vi "通讯.vi"() -> ()   [LabVIEW 2016, in "斯坦道氨氮.lvlib"]
uses:
  <vilib>/Utility/config.llb/Write Key (String).vi
  <vilib>/Plasmionique/MB Master/MB_Master/MB_Master.lvclass
  <vilib>/Utility/config.llb/NI_LVConfig.lvlib
  <vilib>/Plasmionique/MB Master/MB Master.lvlib
panel:
  out "测量数据区":T1 {"单位" items=["ug/L", "mg/L", "ppm", "mg/m3", "cm", "ppb", "ug/m3", "%", "nmol/mol", "umol/mol", "MPN/L", "MPN/100ml", "ng/m3", "NTU", "无量纲", "ms/cm", "us/cm", "℃", "mV", "万个/L"]}
  out "状态告警区":u16[](array[numeric])
  out "测量数据区":u16[](array[numeric])
  out "序列号":string
  out "状态告警区":T2
  out "status":bool
  out "关键参数区":T3
  in  "读关键参数区":bool
  in  "读状态告警区":bool
  in  "读测量数据区":bool
  in  "站号":u16(ring) items=["总磷"=1, "氨氮"=3]
  in  "停止":bool
  in  "启动":bool
  in  "控制命令":u16(ring) items=["启动测量"=1, "标样核查"=2, "零点核查"=3, "跨度核查"=4, "空白测试"=5, "平行样测试"=6, "加标回收"=7, "空白校准"=8, "标样校准"=9, "初始化（清洗）"=10, "停止测试"=11, "仪器重启"=12, "校时"=13, "模式设置"=14, "测量间隔设置"=15]
  in  "控制命令参数":u16[](array[numeric]) format="%04xH"
  in  "VISA Resource":refnum<visa-resource-name>
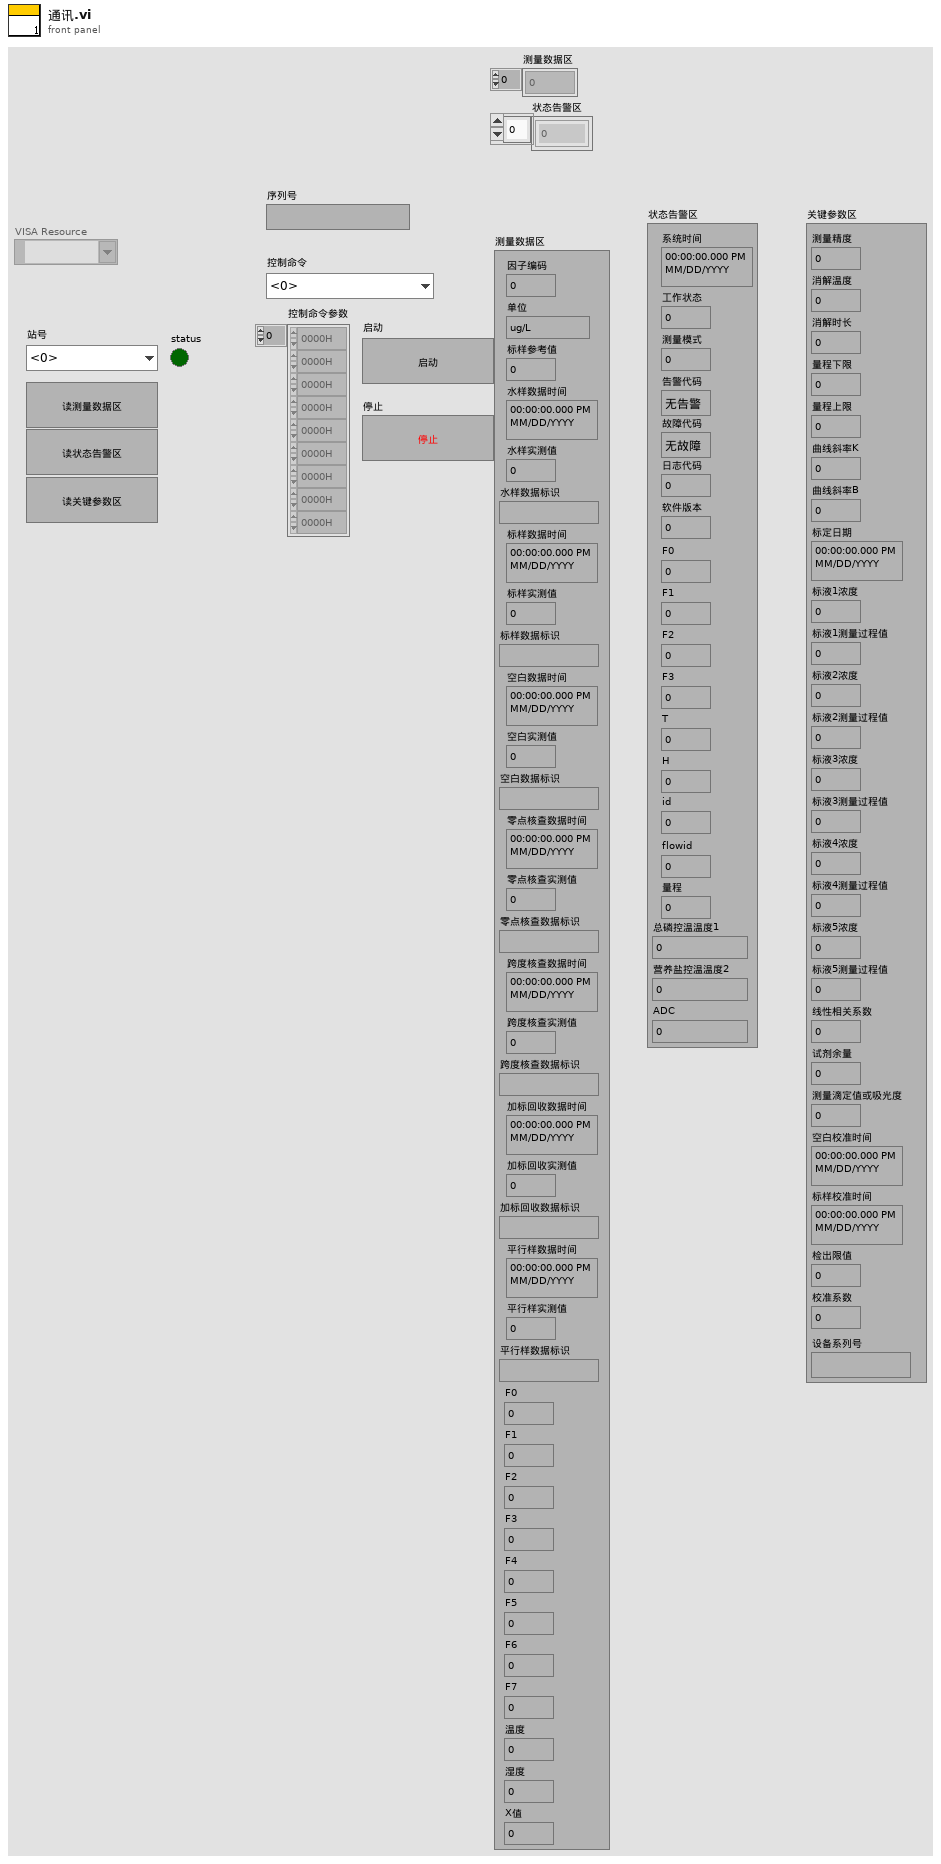
[diagram p1: front panel]
types:
  T1 = cluster{"因子编码":u32, "单位":u16, "标样参考值":sgl, "水样数据时间":timestamp, "水样实测值":sgl, "水样数据标识":string, "标样数据时间":timestamp, "标样实测值":sgl, "标样数据标识":string, "空白数据时间":timestamp, "空白实测值":sgl, "空白数据标识":string, "零点核查数据时间":timestamp, "零点核查实测值":sgl, "零点核查数据标识":string, "跨度核查数据时间":timestamp, "跨度核查实测值":sgl, "跨度核查数据标识":string, "加标回收数据时间":timestamp, "加标回收实测值":sgl, "加标回收数据标识":string, "平行样数据时间":timestamp, "平行样实测值":sgl, "平行样数据标识":string, "F0":sgl, "F1":sgl, "F2":sgl, "F3":sgl, "F4":sgl, "F5":sgl, "F6":sgl, "F7":sgl, "温度":sgl, "湿度":sgl, "X值":sgl}
  T2 = cluster{"系统时间":timestamp, "工作状态":u16, "测量模式":u16, "告警代码":enum16{"无告警", "缺试剂告警", "缺水样告警", "缺蒸馏水告警", "缺标液告警", "仪表漏液告警", "标定异常告警", "超量程告警", "加热异常", "低试剂预警", "超上限告警", "超下限告警", "仪表内部其他异常", "滴定异常告警", "电极异常告警", "量程切换告警", "参数设置告警", "PH电极电位异常", "电导率电极异常", "浊度光度异常", "溶解氧电极异常", "溶解氧光强异常", "温度异常告警", "PH异常告警", "溶解氧异常告警", "电导率异常告警", "浊度异常告警", "叶绿素异常告警", "藻密度异常告警", "蓝绿藻异常告警", "ORP异常告警", "氨氮异常告警", "清洁刷异常告警", "SD卡异常告警", "蓝牙异常告警", "Wifi异常告警", "流程异常告警"}, "故障代码":enum16{"无故障", "电机故障", "温度故障", "通讯故障", "滴定故障"}, "日志代码":u16, "软件版本":u16, "F0":sgl, "F1":sgl, "F2":sgl, "F3":sgl, "T":sgl, "H":sgl, "id":u16, "flowid":u16, "量程":u16, "ADC":sgl, "营养盐控温温度2":sgl, "总磷控温温度1":sgl}
  T3 = cluster{"测量精度":u16, "消解温度":u16, "消解时长":u16, "量程下限":sgl, "量程上限":sgl, "曲线斜率K":sgl, "曲线斜率B":sgl, "标定日期":timestamp, "标液1浓度":sgl, "标液1测量过程值":sgl, "标液2浓度":sgl, "标液2测量过程值":sgl, "标液3浓度":sgl, "标液3测量过程值":sgl, "标液4浓度":sgl, "标液4测量过程值":sgl, "标液5浓度":sgl, "标液5测量过程值":sgl, "线性相关系数":sgl, "试剂余量":u32, "测量滴定值或吸光度":sgl, "空白校准时间":timestamp, "标样校准时间":timestamp, "检出限值":sgl, "校准系数":sgl, "设备系列号":string}
  T4 = typedef "NI_LVConfig.lvlib/Config Data RefNum.ctl" = refnum<k1>
  T5 = enum8{"Enabled", "Disabled", "Disabled and Grayed Out"}
  T6 = cluster{"系统时间":timestamp, "工作状态":enum16{"空闲", "水样测试", "标样核查", "零点核查", "跨度核查", "空白测试", "平行样测试", "加标回收", "空白校准", "标样校准", "初始化（清洗）"}, "测量模式":enum16{"待机", "连续模式", "周期模式", "定点模式", "受控模式", "手动模式"}, "告警代码":enum16{"无告警", "缺试剂告警", "缺水样告警", "缺蒸馏水告警", "缺标液告警", "仪表漏液告警", "标定异常告警", "超量程告警", "加热异常", "低试剂预警", "超上限告警", "超下限告警", "仪表内部其他异常", "滴定异常告警", "电极异常告警", "量程切换告警", "参数设置告警", "PH电极电位异常", "电导率电极异常", "浊度光度异常", "溶解氧电极异常", "溶解氧光强异常", "温度异常告警", "PH异常告警", "溶解氧异常告警", "电导率异常告警", "浊度异常告警", "叶绿素异常告警", "藻密度异常告警", "蓝绿藻异常告警", "ORP异常告警", "氨氮异常告警", "清洁刷异常告警", "SD卡异常告警", "蓝牙异常告警", "Wifi异常告警", "流程异常告警"}, "故障代码":enum16{"无故障", "电机故障", "温度故障", "通讯故障", "滴定故障"}, "日志代码":u16, "软件版本":u16, "F0":sgl, "F1":sgl, "F2":sgl, "F3":sgl, "T":sgl, "H":sgl, "id":u16, "flowid":u16, "量程":u16, "总磷控温温度1":sgl, "营养盐控温温度2":sgl, "ADC":sgl}
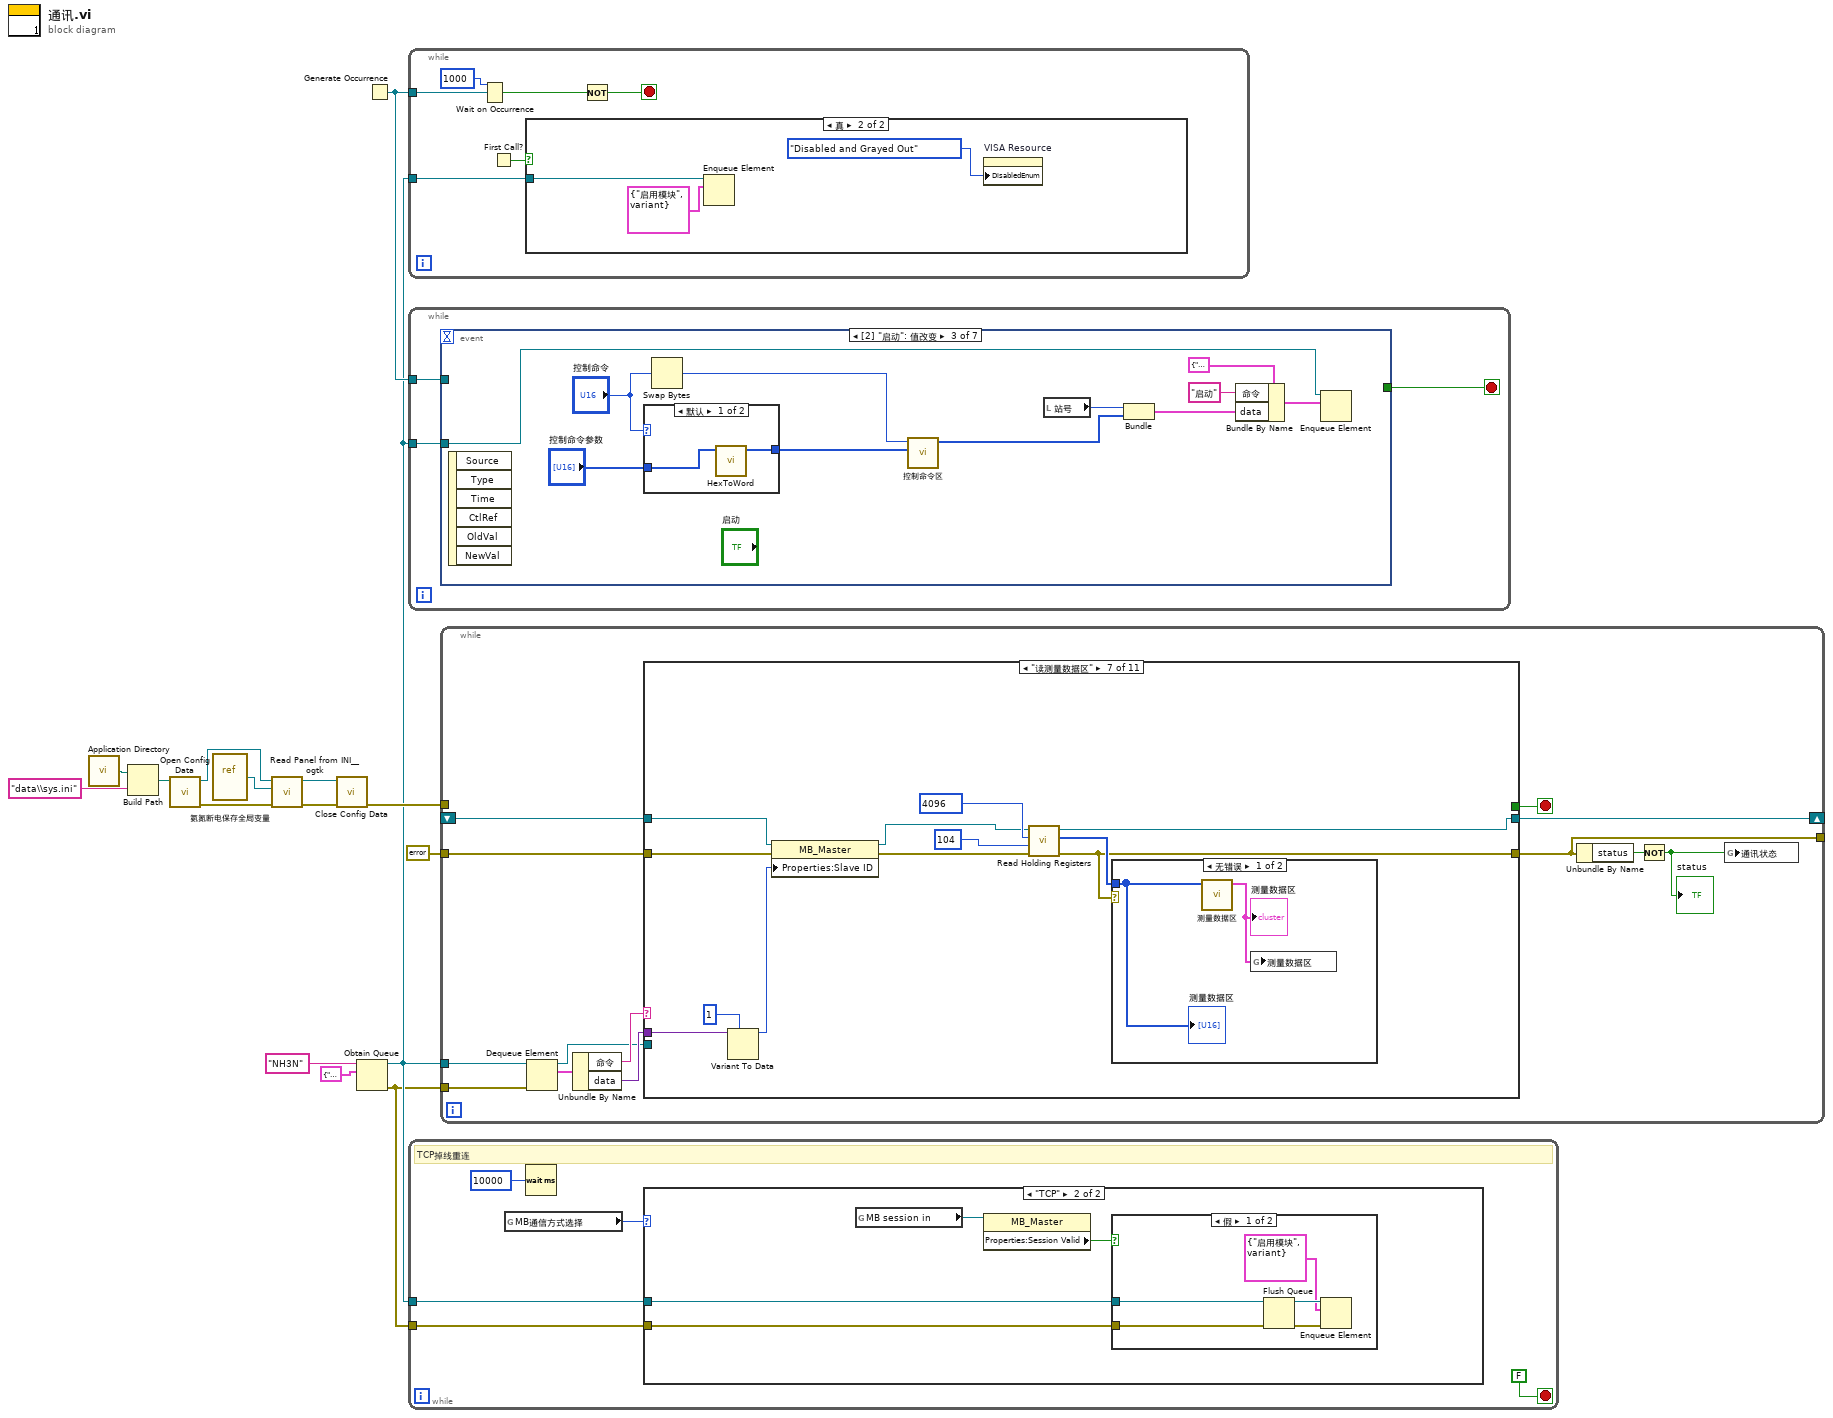
[diagram p0: block diagram]
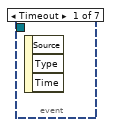
[diagram p5: hidden frame]
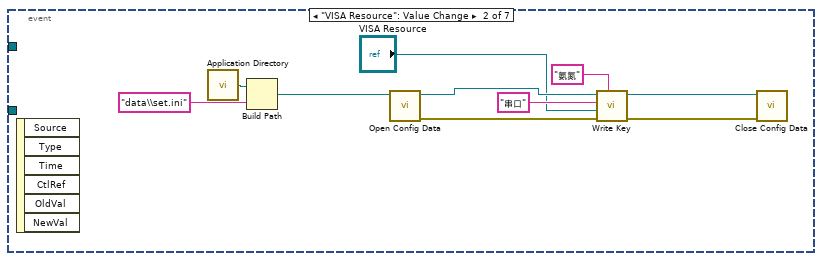
[diagram p6: hidden frame]
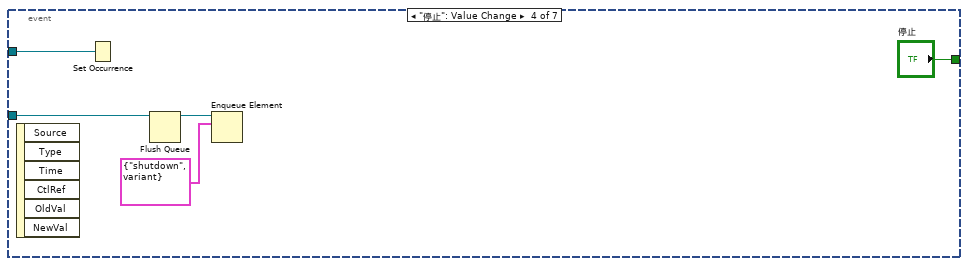
[diagram p8: hidden frame]
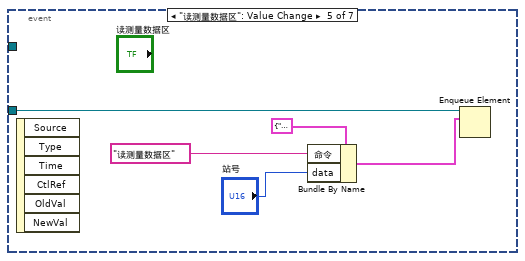
[diagram p9: hidden frame]
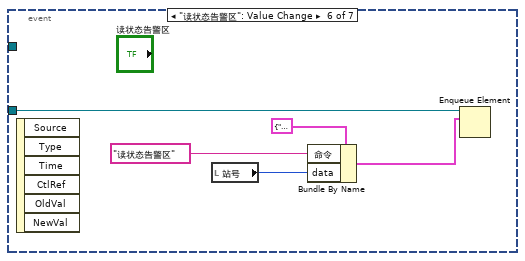
[diagram p10: hidden frame]
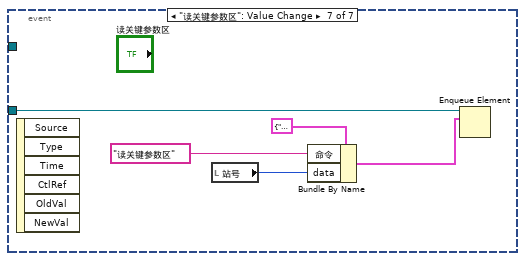
[diagram p11: hidden frame]
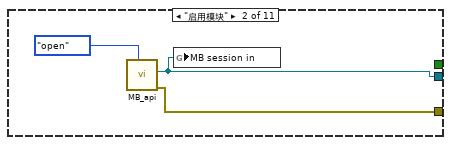
[diagram p13: hidden frame]
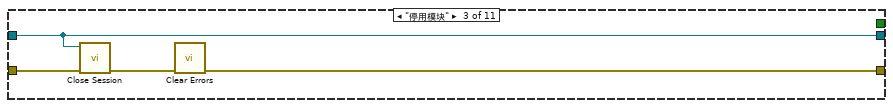
[diagram p14: hidden frame]
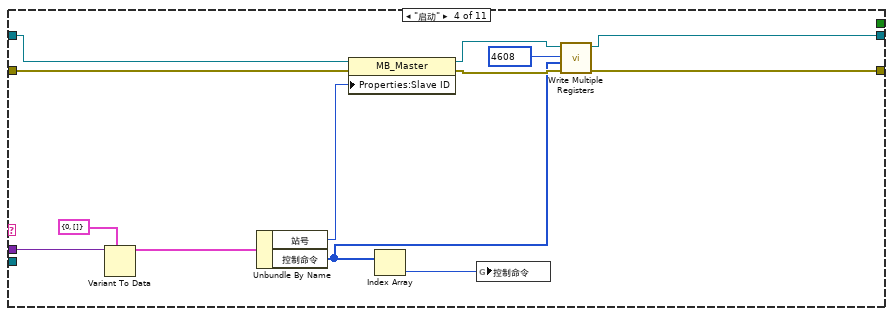
[diagram p15: hidden frame]
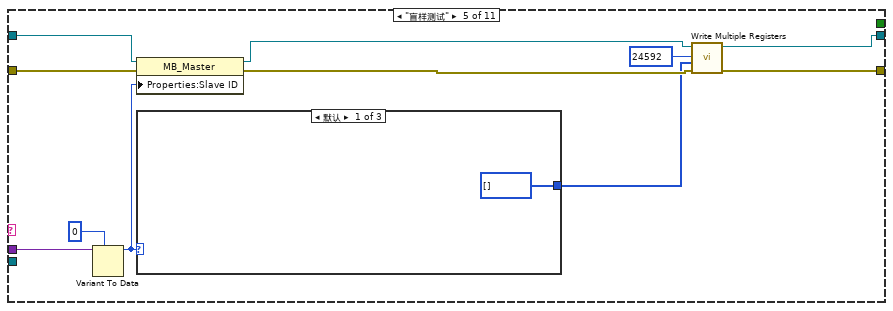
[diagram p16: hidden frame]
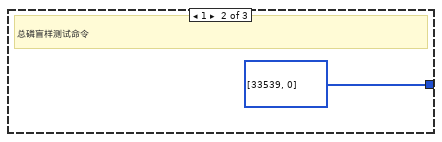
[diagram p17: hidden frame]
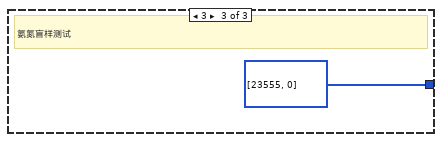
[diagram p18: hidden frame]
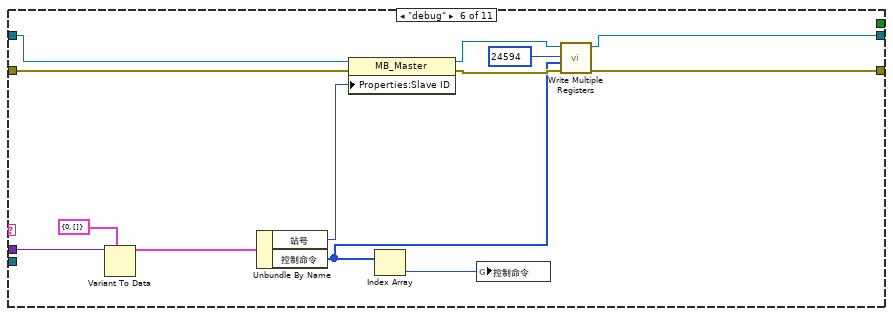
[diagram p19: hidden frame]
diagram:
  n1 = call <vilib>:"Application Directory.vi"() -> ("Application Directory"=w4:path)
  n2 = Build Path(base path=w4, name or relative path="data\\sys.ini" ("名称或相对路径")) -> (appended path=w6:path)
  n3 = call <vilib>:"Open Config Data.vi"("configuration file path"=w6) -> ("error out"=w10:errorcluster, "refnum"=w7:T4)  [unwired: 8 in, 1 out]
  n4 = vi-ref "氨氮断电保存全局变量.vi"() -> (w8:refnum<vi>)
  n5 = call <userlib>:"Read Panel from INI__ogtk.vi"("error in (no error)"=w10, "VI ref"=w8, "refnum"=w7) -> ("error out"=w11:errorcluster, "refnum out"=w9:T4)  [unwired: 7 in]
  n6 = call <vilib>:"Close Config Data.vi"("error in (no error)"=w11, "refnum"=w9) -> ("error out"=w3:errorcluster)  [unwired: 8 in, 1 out]
  n7 = Obtain Queue(name (unnamed)="NH3N" ("名称（未命名）"), element data type=cluster{"命令":string, "data":variant} {"命令"="", "data"=variant}) -> (queue out=w2:refnum<queue>, error out=w1:errorcluster)  [unwired: 3 in, 1 out]
  n8 = Generate Occurrence() -> (w12:refnum<k4>)
  n9 = while {
    tunnel: w12 -> [w21]
    tunnel: w2 -> [w17]
    stop <- w18 stop-if-true
    n10 = Wait on Occurrence(2:w21, 3:1000 ("毫秒超时(-1)")) -> (0:w19:bool)  [unwired: 1 in]
    n11 = First Call?() -> (First Call?: T/F=w16:bool)
    n12 = case shown="真" w16 {
      tunnel: w17 -> [_ w23]
      frame False {
      }
      frame True {
        n13 = Enqueue Element(queue=w23, element=cluster{"命令":string, "data":variant} {"命令"="启用模块", "data"=variant} ("元素")) -> ()  [unwired: 2 in, 3 out]
        n14 = property on="VISA Resource" class="VISAName"("DisabledEnum"=T5."Disabled and Grayed Out" ("禁用")) -> ()  [unwired: 2 in, 2 out]
      }
    }
    n15 = Not(x=w19) -> (.not. x?=w18:bool)
  }
  n16 = while {
    tunnel: w2 -> [w27]
    tunnel: w12 -> [w25]
    stop <- w26 stop-if-true
    n17 = event shown="[2] \"启动\": 值改变" {
      selector: _ -> [_ _ _ _ _ _ _]
      dyn-events: _ -> [_ _ _ _ _ _ _]
      timeout: _ -> [_ _ _ _ _ _ _]
      tunnel: w27 -> [_ _ w48 w55 w61 w66 w71]
      tunnel: [_ _ _ "停止" _ _ _] -> w26
      tunnel: w25 -> [_ _ _ w52 _ _ _]
      event Timeout {
        n18 = event-data() -> ()  [unwired: 1 in, 3 out]
      }
      event "VISA Resource": Value Change {
        n19 = event-data() -> ()  [unwired: 1 in, 6 out]
        n20 = call <vilib>:"Application Directory.vi"() -> ("Application Directory"=w30:path)
        n21 = Build Path(base path=w30, name or relative path="data\\set.ini" ("名称或相对路径")) -> (appended path=w31:path)
        n22 = call <vilib>:"Open Config Data.vi"("configuration file path"=w31) -> ("error out"=w37:errorcluster, "refnum"=w36:T4)  [unwired: 8 in, 1 out]
        n23 = call-poly <vilib>:"Write Key.vi"("section"="氨氮", "error in (no error)"=w37, "value"="VISA Resource", "key"="串口", "refnum"=w36) -> ("error out"=w33:errorcluster, "refnum out"=w29:T4)  [unwired: 4 in, 1 out]
        n24 = call <vilib>:"Close Config Data.vi"("error in (no error)"=w33, "refnum"=w29) -> ()  [unwired: 8 in, 2 out]
      }
      event "启动": Value Change {
        n25 = event-data() -> ()  [unwired: 1 in, 6 out]
        n26 = case shown="默认" "控制命令" {
          tunnel: "控制命令参数" -> [w50 w51]
          tunnel: [w49 w51] -> w38
          frame Default {
            n27 = call "HexToWord.vi"("数组"=w50) -> ("WORD"=w49:u16[])  [unwired: 10 in]
          }
          frame 13 {
          }
        }
        n28 = Swap Bytes(anything="控制命令") -> (byte swapped=w41:u16)
        n29 = call "控制命令区.vi"("控制命令参数"=w38, "控制命令"=w41) -> ("控制命令"=w44:u16[])  [unwired: 9 in]
        n30 = local read "站号"() -> (w43:u16)
        n31 = Bundle("站号"=w43, "控制命令"=w44) -> (w42:cluster{"站号":u16, "控制命令":u16[]})  [unwired: 1 in]
        n32 = Bundle By Name(cluster=cluster{"命令":string, "data":variant} {"命令"="", "data"=variant} ("元素"), "命令"="启动", "data"=w42) -> (w46:cluster{"命令":string, "data":variant})
        n33 = Enqueue Element(queue=w48, element=w46) -> ()  [unwired: 2 in, 3 out]
      }
      event "停止": Value Change {
        n34 = event-data() -> ()  [unwired: 1 in, 6 out]
        n35 = Set Occurrence(w52) -> ()
        n36 = Flush Queue(queue=w55) -> (queue out=w54:refnum<queue>)  [unwired: 1 in, 2 out]
        n37 = Enqueue Element(queue=w54, element=cluster{"命令":string, "data":variant} {"命令"="shutdown", "data"=variant} ("元素")) -> ()  [unwired: 2 in, 3 out]
      }
      event "读测量数据区": Value Change {
        n38 = event-data() -> ()  [unwired: 1 in, 6 out]
        n39 = Bundle By Name(cluster=cluster{"命令":string, "data":variant} {"命令"="", "data"=variant} ("元素"), "命令"="读测量数据区", "data"="站号") -> (w59:cluster{"命令":string, "data":variant})
        n40 = Enqueue Element(queue=w61, element=w59) -> ()  [unwired: 2 in, 3 out]
      }
      event "读状态告警区": Value Change {
        n41 = event-data() -> ()  [unwired: 1 in, 6 out]
        n42 = local read "站号"() -> (w62:u16)
        n43 = Bundle By Name(cluster=cluster{"命令":string, "data":variant} {"命令"="", "data"=variant} ("元素"), "命令"="读状态告警区", "data"=w62) -> (w64:cluster{"命令":string, "data":variant})
        n44 = Enqueue Element(queue=w66, element=w64) -> ()  [unwired: 2 in, 3 out]
      }
      event "读关键参数区": Value Change {
        n45 = event-data() -> ()  [unwired: 1 in, 6 out]
        n46 = local read "站号"() -> (w67:u16)
        n47 = Bundle By Name(cluster=cluster{"命令":string, "data":variant} {"命令"="", "data"=variant} ("元素"), "命令"="读关键参数区", "data"=w67) -> (w69:cluster{"命令":string, "data":variant})
        n48 = Enqueue Element(queue=w71, element=w69) -> ()  [unwired: 2 in, 3 out]
      }
    }
  }
  n49 = while "While循环" {
    tunnel: w2 -> [w74]
    tunnel: w1 -> [w73]
    stop <- FALSE stop-if-true
    # "TCP掉线重连"
    n50 = global read "氨氮断电保存全局变量.vi" "MB通信方式选择"() -> (w72:enum16{"串口", "TCP"})
    n51 = Wait (ms)(milliseconds to wait=u32 10000 ("等待时间（毫秒）")) -> ()  [unwired: 1 out]
    n52 = case shown="\"TCP\"" w72 {
      tunnel: w74 -> [_ w79]
      tunnel: w73 -> [_ w78]
      frame "串口", Default {
      }
      frame "TCP" {
        n53 = global read "VAR氨氮全局变量.vi" "MB session in"() -> (w77:refnum<class "MB_Master.lvclass">)
        n54 = property class="MB_Master"(reference=w77) -> ("Properties:Session Valid"=w80:bool)  [unwired: 1 in, 2 out]
        n55 = case shown="假" w80 {
          tunnel: w79 -> [w83 _]
          tunnel: w78 -> [w82 _]
          frame False {
            n56 = Flush Queue(queue=w83, error in (no error)=w82) -> (queue out=w85:refnum<queue>, error out=w84:errorcluster)  [unwired: 1 out]
            n57 = Enqueue Element(queue=w85, element=cluster{"命令":string, "data":variant} {"命令"="启用模块", "data"=variant} ("元素"), error in (no error)=w84) -> ()  [unwired: 1 in, 3 out]
          }
          frame True {
          }
        }
      }
    }
  }
  n58 = while {
    tunnel: w2 -> [w98]
    tunnel: w1 -> [w97]
    shift-right: [w95] -> _
    shift-left: _ -> [w94]
    tunnel: errorcluster {"status"=FALSE, "code"=0, "source"=""} ("error out") -> [w93]
    tunnel: [w88] -> _
    tunnel: w3 -> [_]
    stop <- w96 stop-if-true
    n59 = Dequeue Element(queue=w98, error in (no error)=w97) -> (queue out=w89:refnum<queue>, element=w91:cluster{"命令":string, "data":variant})  [unwired: 1 in, 2 out]
    n60 = Unbundle By Name(w91) -> ("命令"=w92:string, "data"=w90:variant)
    n61 = case shown="\"读测量数据区\"" w92 {
      tunnel: w90 -> [_ _ _ w117 w128 w145 w154 w164 w179 w193 _]
      tunnel: w89 -> [_ _ _ _ _ _ _ _ _ _ w206]
      tunnel: [_ _ _ _ _ _ _ _ _ _ TRUE] -> w96
      tunnel: [w99 w102 w104 w120 w131 w147 w159 w173 w186 w200 w202] -> w95
      tunnel: [w100 w101 w105 w119 w130 w146 w148 w174 w187 w201 w203] -> w88
      tunnel: w94 -> [w99 _ w104 w116 w127 w144 w153 w167 w182 w196 w202]
      tunnel: w93 -> [w100 _ w107 w113 w124 w141 w151 w168 w183 w197 w204]
      frame Default {
      }
      frame "启用模块" {
        n62 = call "MB_api.vi"("STEP"=enum16{"open", "read", "write", "close"}."open") -> ("error out"=w101:errorcluster, "MB session out"=w102:refnum<class "MB_Master.lvclass">)  [unwired: 8 in, 1 out]
        n63 = global write "VAR氨氮全局变量.vi" "MB session in"(w102) -> ()
      }
      frame "停用模块" {
        n64 = call-dynamic "Close Session.vi"("error in (no error)"=w107, "MB session in"=w104) -> ("error out"=w106:errorcluster)  [unwired: 9 in]
        n65 = call <vilib>:"Clear Errors.vi"("error in (no error)"=w106) -> ("error out"=w105:errorcluster)  [unwired: 5 in, 1 out]
      }
      frame "启动" {
        n66 = Variant To Data(type=cluster{"站号":u16, "控制命令":u16[]} {"站号"=0, "控制命令"=[]} ("输出簇"), Variant=w117) -> (data=w111:cluster{"站号":u16, "控制命令":u16[]})  [unwired: 1 in, 1 out]
        n67 = Unbundle By Name(w111) -> ("站号"=w110:u16, "控制命令"=w108:u16[])
        n68 = property class="MB_Master"(reference=w116, error in=w113, "Properties:Slave ID"=w110) -> (reference out=w115:refnum<class "MB_Master.lvclass">, error out=w114:errorcluster)
        n69 = Index Array(array=w108) -> (element=w109:u16)  [unwired: 1 in]
        n70 = global write "VAR氨氮全局变量.vi" "控制命令"(w109) -> ()
        n71 = call <vilib>:"Write Multiple Registers.vi"("error in (no error)"=w114, "values"=w108, "starting address"=u16 4608, "MB session in"=w115) -> ("error out"=w119:errorcluster, "MB session out"=w120:refnum<class "MB_Master.lvclass">)  [unwired: 6 in]
      }
      frame "盲样测试" {
        n72 = Variant To Data(type=0, Variant=w128) -> (data=w121:i32)  [unwired: 1 in, 1 out]
        n73 = property class="MB_Master"(reference=w127, error in=w124, "Properties:Slave ID"=w121) -> (reference out=w126:refnum<class "MB_Master.lvclass">, error out=w125:errorcluster)
        n74 = case shown="默认" w121 {
          tunnel: [u16[] [] ("values") u16[] [33539, 0] ("values") u16[] [23555, 0] ("values")] -> w123
          frame Default {
          }
          frame 1 {
            # "总磷盲样测试命令"
          }
          frame 3 {
            # "氨氮盲样测试"
          }
        }
        n75 = call <vilib>:"Write Multiple Registers.vi"("error in (no error)"=w125, "values"=w123, "starting address"=u16 24592, "MB session in"=w126) -> ("error out"=w130:errorcluster, "MB session out"=w131:refnum<class "MB_Master.lvclass">)  [unwired: 6 in]
      }
      frame "debug" {
        n76 = Variant To Data(type=cluster{"站号":u16, "控制命令":u16[]} {"站号"=0, "控制命令"=[]} ("输出簇"), Variant=w145) -> (data=w139:cluster{"站号":u16, "控制命令":u16[]})  [unwired: 1 in, 1 out]
        n77 = Unbundle By Name(w139) -> ("站号"=w138:u16, "控制命令"=w136:u16[])
        n78 = property class="MB_Master"(reference=w144, error in=w141, "Properties:Slave ID"=w138) -> (reference out=w143:refnum<class "MB_Master.lvclass">, error out=w142:errorcluster)
        n79 = Index Array(array=w136) -> (element=w137:u16)  [unwired: 1 in]
        n80 = global write "VAR氨氮全局变量.vi" "控制命令"(w137) -> ()
        n81 = call <vilib>:"Write Multiple Registers.vi"("error in (no error)"=w142, "values"=w136, "starting address"=u16 24594, "MB session in"=w143) -> ("error out"=w146:errorcluster, "MB session out"=w147:refnum<class "MB_Master.lvclass">)  [unwired: 6 in]
      }
      frame "读测量数据区" {
        n82 = Variant To Data(type=u8 1 ("Slave ID"), Variant=w154) -> (data=w155:u8)  [unwired: 1 in, 1 out]
        n83 = property class="MB_Master"(reference=w153, error in=w151, "Properties:Slave ID"=w155) -> (reference out=w152:refnum<class "MB_Master.lvclass">, error out=w150:errorcluster)
        n84 = call <vilib>:"Read Holding Registers.vi"("error in (no error)"=w150, "quantity"=u16 104, "starting address"=u16 4096, "MB session in"=w152) -> ("error out"=w148:errorcluster, "Registers"=w149:u16[], "MB session out"=w159:refnum<class "MB_Master.lvclass">)  [unwired: 5 in]
        n85 = case shown="无错误" w148 {
          tunnel: w149 -> [w161 _]
          frame No Error {
            n86 = call "测量数据区.vi"("数组"=w161) -> ("测量数据区"=w160:T1)  [unwired: 10 in]
            "测量数据区" <- w160
            n87 = global write "VAR氨氮全局变量.vi" "测量数据区"(w160) -> ()
            "测量数据区" <- w161
          }
          frame Error {
          }
        }
      }
      frame "读状态告警区" {
        n88 = Variant To Data(type=u8 1 ("Slave ID"), Variant=w164) -> (data=w169:u8)  [unwired: 1 in, 1 out]
        n89 = property class="MB_Master"(reference=w167, error in=w168, "Properties:Slave ID"=w169) -> (reference out=w166:refnum<class "MB_Master.lvclass">, error out=w165:errorcluster)
        n90 = call <vilib>:"Read Holding Registers.vi"("error in (no error)"=w165, "quantity"=u16 24, "starting address"=u16 4224, "MB session in"=w166) -> ("error out"=w174:errorcluster, "Registers"=w163:u16[], "MB session out"=w173:refnum<class "MB_Master.lvclass">)  [unwired: 5 in]
        "状态告警区" <- w163
        n91 = call "状态告警区.vi"("数组"=w163) -> ("状态告警区"=w162:T6)  [unwired: 10 in]
        "状态告警区" <- w162
        n92 = global write "VAR氨氮全局变量.vi" "状态告警区"(w162) -> ()
      }
      frame "读关键参数区" {
        n93 = Variant To Data(type=u8 1 ("Slave ID"), Variant=w179) -> (data=w177:u8)  [unwired: 1 in, 1 out]
        n94 = property class="MB_Master"(reference=w182, error in=w183, "Properties:Slave ID"=w177) -> (reference out=w181:refnum<class "MB_Master.lvclass">, error out=w180:errorcluster)
        n95 = call <vilib>:"Read Holding Registers.vi"("error in (no error)"=w180, "quantity"=u16 19, "starting address"=u16 4256, "MB session in"=w181) -> ("error out"=w187:errorcluster, "Registers"=w176:u16[], "MB session out"=w186:refnum<class "MB_Master.lvclass">)  [unwired: 5 in]
        n96 = call "关键参数区.vi"("数组"=w176) -> ("关键参数区"=w175:T3)  [unwired: 10 in]
        "关键参数区" <- w175
        n97 = global write "VAR氨氮全局变量.vi" "关键参数区"(w175) -> ()
      }
      frame "读序列号" {
        n98 = Variant To Data(type=u8 1 ("Slave ID"), Variant=w193) -> (data=w191:u8)  [unwired: 1 in, 1 out]
        n99 = property class="MB_Master"(reference=w196, error in=w197, "Properties:Slave ID"=w191) -> (reference out=w195:refnum<class "MB_Master.lvclass">, error out=w194:errorcluster)
        n100 = call <vilib>:"Read Holding Registers.vi"("error in (no error)"=w194, "quantity"=u16 6, "starting address"=u16 3, "MB session in"=w195) -> ("error out"=w201:errorcluster, "Registers"=w190:u16[], "MB session out"=w200:refnum<class "MB_Master.lvclass">)  [unwired: 5 in]
        n101 = call "HexToString.vi"("数组"=w190) -> ("STRING"=w189:string[])  [unwired: 10 in]
        n102 = Index Array(array=w189) -> (element=w188:string)  [unwired: 1 in]
        "序列号" <- w188
        n103 = global write "VAR氨氮全局变量.vi" "序列号"(w188) -> ()
      }
      frame "shutdown" {
        n104 = call-dynamic "Close Session.vi"("error in (no error)"=w204, "MB session in"=w202) -> ("error out"=w203:errorcluster)  [unwired: 9 in]
        n105 = Flush Queue(queue=w206) -> (queue out=w205:refnum<queue>)  [unwired: 1 in, 2 out]
        n106 = Release Queue(queue=w205) -> ()  [unwired: 2 in, 3 out]
      }
    }
    n107 = Unbundle By Name(w88) -> ("status"=w87:bool)
    n108 = Not(x=w87) -> (.not. x?=w86:bool)
    "status" <- w86
    n109 = global write "VAR氨氮全局变量.vi" "通讯状态"(w86) -> ()
  }
